vi "VirtualInstrument.vi"() -> ()   [LabVIEW 2011]
uses:
  <vilib>/Analysis/5stat.llb/RMS (DBL).vi
  <vilib>/Analysis/NI_AALPro.lvlib
panel:
  in  "Arquivo de Saída":path
  in  "Gravar Arquivo":bool
  out "Hora e Data (UTC)":timestamp format="%^<%.3X\n%x>T"
  out "Hora e Data (Local)":timestamp
  out "Tempo":dbl format="%#_13g"
  out "Potência":dbl(graph)
  out "Corrente RMS":dbl(graph)
  out "Tensão RMS":dbl(graph)
  in  "Mult. Corrente":dbl
  out "Corrente Lida":dynamicdata(graph)
  in  "Loop":bool
  out "Tensão Lida":dynamicdata(graph)
  in  "Amostras":dbl
  in  "Frequência":dbl
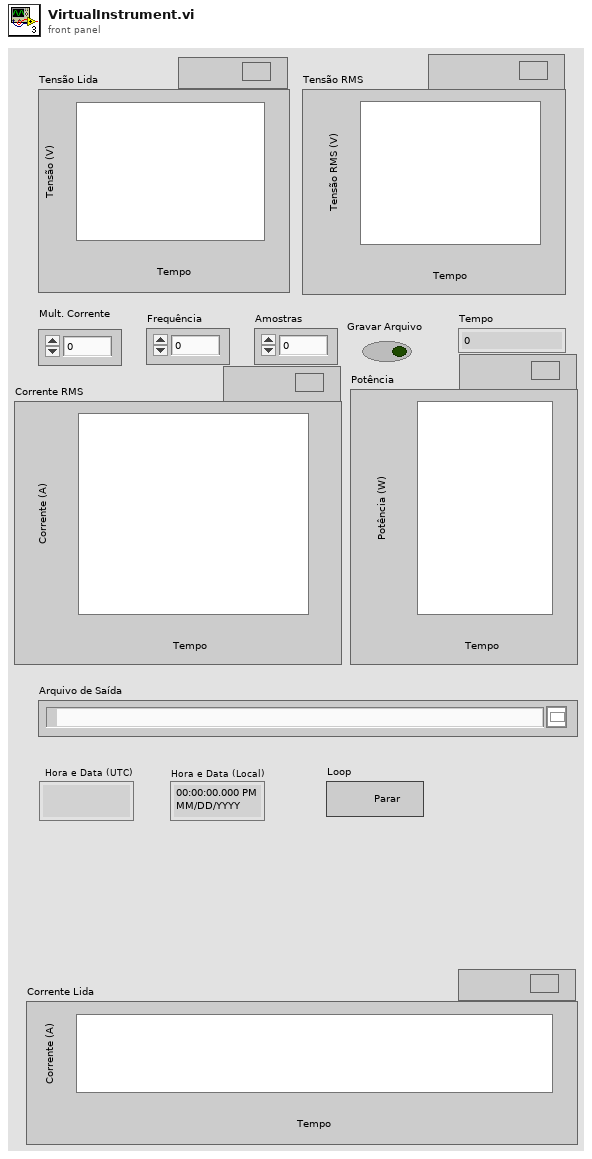
[diagram p1: front panel]
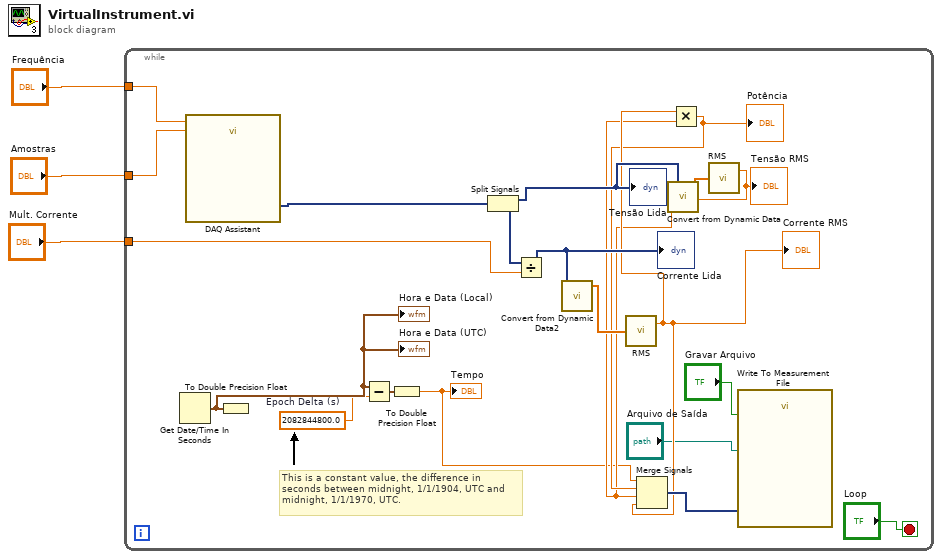
[diagram p0: block diagram]
diagram:
  n1 = while {
    tunnel: "Amostras" -> [w22]
    tunnel: "Frequência" -> [w21]
    tunnel: "Mult. Corrente" -> [w20]
    stop <- "Loop" stop-if-true
    w8 = 2082844800.0  # Epoch Delta (s)
    # "This is a constant value, the difference in seconds between midnight, 1/1/1904, UTC and midnight, 1/1/1970, UTC."
    n2 = Get Date/Time In Seconds() -> (seconds since 1Jan1904=w9:timestamp)
    "Hora e Data (Local)" <- w9
    "Hora e Data (UTC)" <- w9
    n3 = call "DAQ Assistant"("rate"=w21, "number of samples"=w22) -> ("data"=w16:dynamicdata)  [unwired: 15 in, 2 out]
    n4 = To Double Precision Float(number=w9) -> ()  [unwired: 1 out]
    n5 = Subtract(x=w9, y=w8) -> (x-y=w7:timestamp)
    n6 = To Double Precision Float(number=w7) -> (double precision float=w6:dbl)
    "Tempo" <- w6
    n7 = Split Signals(w16) -> (w18:dynamicdata, w19:dynamicdata)  [unwired: 2 in]
    "Tensão Lida" <- w18
    n8 = Divide(x=w19, y=w20) -> (x/y=w15:dynamicdata)
    "Corrente Lida" <- w15
    n9 = call "Convert from Dynamic Data2"("Dynamic Data Type"=w15) -> ("Array"=w14:dbl[])  [unwired: 3 in]
    n10 = call-poly <vilib>:"RMS.vi"("X"=w14) -> ("rms value"=w12:dbl)  [unwired: 1 out]
    "Corrente RMS" <- w12
    n11 = call "Convert from Dynamic Data"("Dynamic Data Type"=w18) -> ("Array"=w17:dbl[])  [unwired: 3 in]
    n12 = call-poly <vilib>:"RMS.vi"("X"=w17) -> ("rms value"=w10:dbl)  [unwired: 1 out]
    "Tensão RMS" <- w10
    n13 = Multiply(x=w12, y=w10) -> (x*y=w11:dbl)
    "Potência" <- w11
    n14 = Merge Signals(w6, w11, w10, w12) -> (w13:dynamicdata)
    n15 = call "Write To Measurement File"("Signals"=w13, "Enable"="Gravar Arquivo", "Filename"="Arquivo de Saída") -> ()  [unwired: 14 in, 3 out]
  }
